vi "CreatePXI6229Tasks.vi"(8 "Error In":errorcluster) -> (0 "Error Out":errorcluster, 3 "PXI-6229 Tasks Out":refnum<k21>[](array[refnum]))   [LabVIEW 2012]
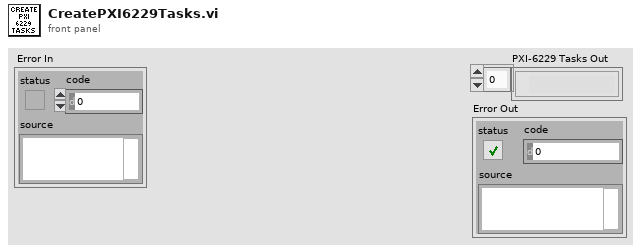
[diagram p1: front panel]
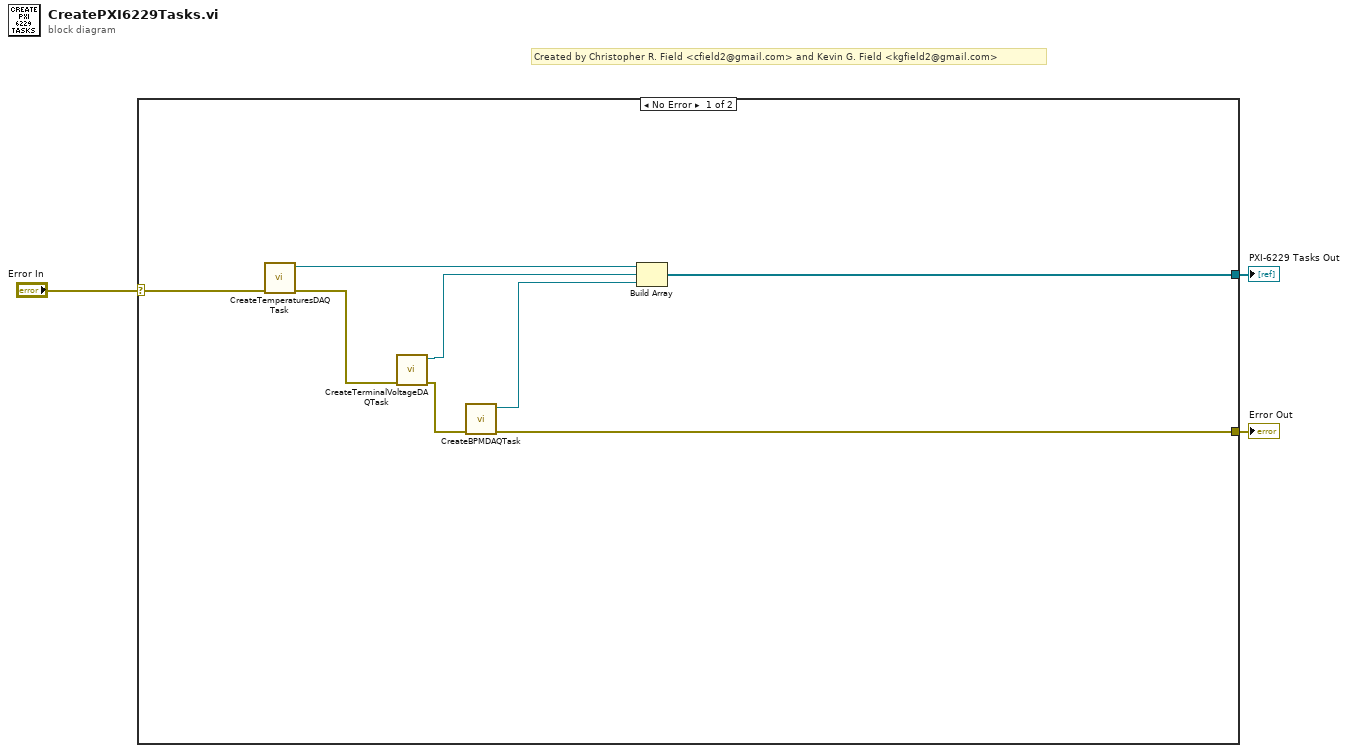
[diagram p0: block diagram]
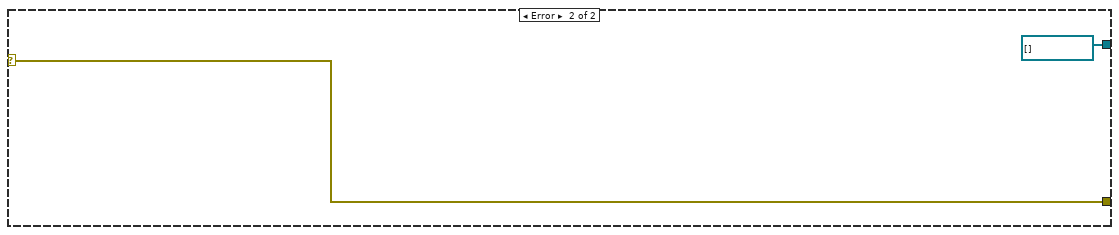
[diagram p2: hidden frame]
diagram:
  # "Created by Christopher R. Field <cfield2@gmail.com> and Kevin G. Field <kgfield2@gmail.com>"
  n1 = case shown="No Error" "Error In" {
    selector: "Error In" -> [w9 w13]
    tunnel: [w10 w13] -> w1
    tunnel: [w7 refnum<k21>[] []] -> w2
    frame No Error {
      n2 = call "CreateTemperaturesDAQTask.vi"("Error In"=w9) -> ("Error Out"=w4:errorcluster, "Temperatures Task"=w8:refnum<k21>)  [unwired: 9 in]
      n3 = call "CreateTerminalVoltageDAQTask.vi"("Error In"=w4) -> ("Error Out"=w11:errorcluster, "Terminal Voltage Task"=w6:refnum<k21>)  [unwired: 9 in]
      n4 = call "CreateBPMDAQTask.vi"("Error In"=w11) -> ("Error Out"=w10:errorcluster, "BPM Task"=w5:refnum<k21>)  [unwired: 9 in]
      n5 = Build Array(w8, w6, w5) -> (w7:refnum<k21>[])
    }
    frame Error {
    }
  }
  "PXI-6229 Tasks Out" <- w2
  "Error Out" <- w1
